vi "serial12.vi"() -> ()   [LabVIEW 2019]
uses:
  <vilib>/Instr/_visa.llb/VISA Configure Serial Port (Instr).vi
panel:
  out "Boolean":bool
  out "Estado":bool
  in  "Guardar Config":bool
  in  "Detener":bool
  in  "Iniciar":bool
  in  "Puerto Comunicación":refnum<visa-resource-name>
  out "Presión Instantánea":dbl[unit]
  out "Velocidad Turbina %":dbl[unit]
  in  "Presión Tope":dbl
  in  "PEEP":dbl
  in  "Tiempo Meseta":dbl
  in  "Turbina %":dbl
  out "XY Graph":cluster{"X":dbl, "Y":dbl}[](graph)
  out "Waveform Chart":dbl(graph)
  in  "WRITE":bool
  in  "write buffer":string
  in  "stop":bool
  out "read buffer":string
  in  "READ":bool
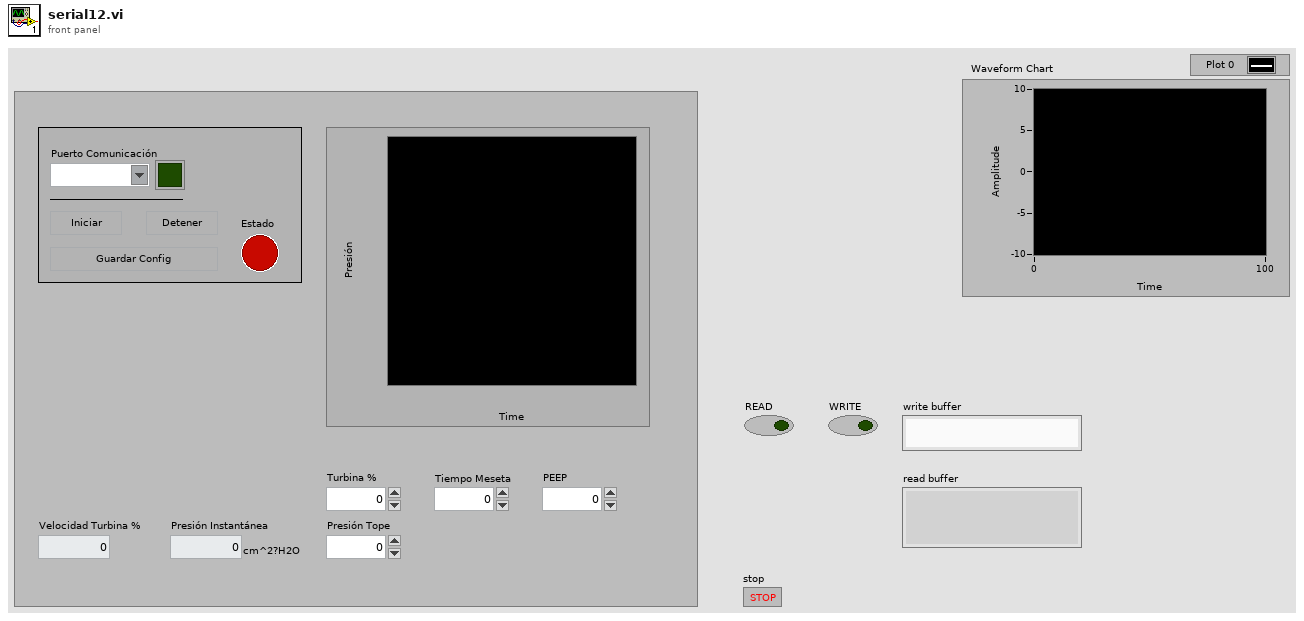
[diagram p1: front panel]
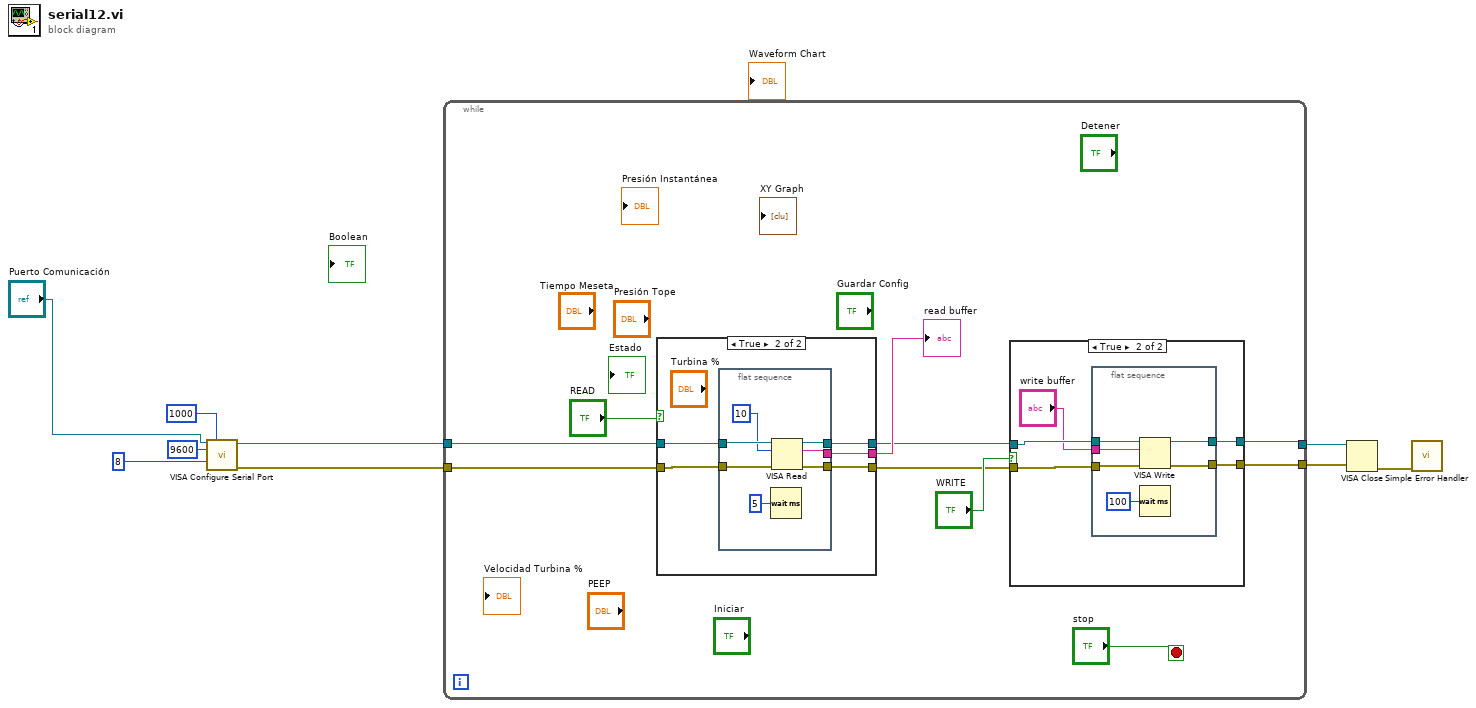
[diagram p0: block diagram]
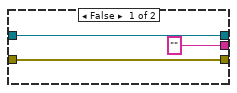
[diagram p3: hidden frame]
diagram:
  n1 = call-poly "VISA Configure Serial Port"("VISA resource name"="Puerto Comunicación", "timeout (10sec)"=u32 1000, "baud rate (9600)"=u32 9600, "data bits (8)"=u16 8) -> ("VISA resource name out"=w8:refnum<visa-resource-name>, "error out"=w7:errorcluster)  [unwired: 5 in, 5 out]
  n2 = while {
    tunnel: w8 -> [w16]
    tunnel: w7 -> [w14]
    tunnel: [w11] -> w4
    tunnel: [w10] -> w3
    stop <- "stop" stop-if-true
    n3 = case shown="True" "READ" {
      tunnel: w16 -> [w35 w40]
      tunnel: w14 -> [w34 w39]
      tunnel: [w35 w37] -> w13
      tunnel: [w34 w38] -> w12
      tunnel: ["" ("read buffer") w36] -> w18
      frame False {
      }
      frame True {
        n4 = flat-sequence {
          tunnel: w40 -> [w47]
          tunnel: w39 -> [w46]
          tunnel: [w45] -> w37
          tunnel: [w44] -> w38
          tunnel: [w43] -> w36
          frame #0 {
            n5 = Wait (ms)(milliseconds to wait=u32 5) -> ()  [unwired: 1 out]
            n6 = VISA Read(VISA resource name=w47, byte count=u32 10, error in (no error)=w46) -> (VISA resource name out=w45:refnum<visa-resource-name>, read buffer=w43:string, error out=w44:errorcluster)  [unwired: 1 out]
          }
        }
      }
    }
    "read buffer" <- w18
    n7 = case shown="True" "WRITE" {
      tunnel: w13 -> [w21 w26]
      tunnel: w12 -> [w20 w25]
      tunnel: [w21 w23] -> w11
      tunnel: [w20 w22] -> w10
      frame False {
      }
      frame True {
        n8 = flat-sequence {
          tunnel: w26 -> [w32]
          tunnel: w25 -> [w31]
          tunnel: "write buffer" -> [w30]
          tunnel: [w29] -> w23
          tunnel: [w28] -> w22
          frame #0 {
            n9 = VISA Write(VISA resource name=w32, write buffer=w30, error in (no error)=w31) -> (VISA resource name out=w29:refnum<visa-resource-name>, error out=w28:errorcluster)  [unwired: 1 out]
            n10 = Wait (ms)(milliseconds to wait=u32 100) -> ()  [unwired: 1 out]
          }
        }
      }
    }
  }
  n11 = VISA Close(VISA resource name=w4, error in (no error)=w3) -> (error out=w9:errorcluster)
  n12 = call <vilib>:"Simple Error Handler.vi"("error in (no error)"=w9) -> ()  [unwired: 1 in, 8 out]
